vi "MSScript_SubVI_UpdataColour.vi"(7 "TextProperties":T1={"Colour"=16711680, "Italic"=FALSE, "Bold"=FALSE}, 9 "CMNT in":cluster{"Start":u32, "End":u32}[](array[cluster]), 10 "Expression.Section":cluster{"STR":string, "Start":i32}, 11 "String ref in":refnum<vi>) -> ()   [LabVIEW 2018, in "MSScript.lvclass"]
uses:
  MSScript.lvclass
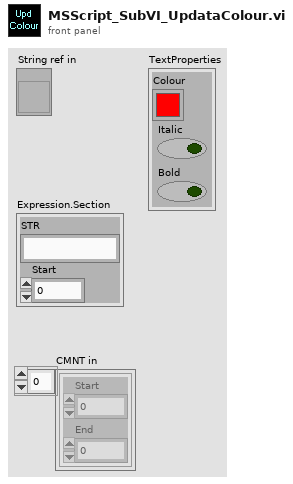
[diagram p1: front panel]
types:
  T1 = cluster{"Colour":u32, "Italic":bool, "Bold":bool}
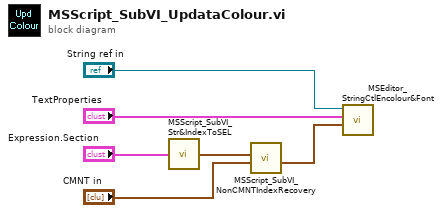
[diagram p0: block diagram]
diagram:
  n1 = call "MSScript_SubVI_Str&IndexToSEL.vi"("Name string"="Expression.Section") -> ("SEL"=w5:cluster{"Start":u32, "End":u32}[])
  n2 = call "MSScript_SubVI_NonCMNTIndexRecovery.vi"("SEL of CMNT"="CMNT in", "NonCMNT.SEL"=w5) -> ("RecoverySEL"=w6:cluster{"Start":u32, "End":u32}[])  [unwired: 5 in]
  n3 = call "MSEditor_StringCtlEncolour&Font.vi"("SELs"=w6, "TextProperties"="TextProperties", "String ctl ref"="String ref in") -> ()  [unwired: 7 in, 2 out]
